vi "Modify Channel Test.vi"() -> (0 "no err":errorcluster, 3 "mod success":bool)   [LabVIEW 2017, in "ExampleStateMachine tests.lvlib"]
uses:
  ExampleStateMachine tests.lvlib
  <vilib>/NI/Tag Bus Module Framework/channel/TBM channel.lvclass/TBM channel.ctl
  <vilib>/NI/Tag Bus Module Framework/channel/channel classification.ctl
  <vilib>/NI/Tag Bus/tag/tag descriptor.lvclass/tag descriptor.ctl
  <vilib>/NI/Tag Bus Module Framework/channel/Read channel classification.vi
  <vilib>/NI/Tag Bus Module Framework/channel/Write channel classification.vi
  <vilib>/NI/Tag Bus Module Framework/channel/TBM channel.lvclass
  C:/Program Files (x86)/National Instruments/LabVIEW 2017/vi.lib/NI/Tag Bus/tag/tag descriptor.lvclass
  module/configuration/ExampleStateMachine configuration.lvclass
  <vilib>/NI/Tag Bus/tag/tag descriptor.lvclass
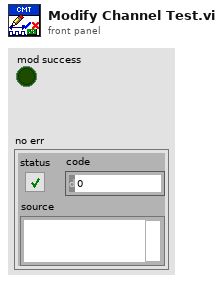
[diagram p1: front panel]
types:
  T1 = cluster{"channel":refnum<class "TBM channel.lvclass">}[]
  T2 = typedef "TBM channel.lvclass/channel classification.ctl" = enum16{"input data", "output data", "processing parameter", "processing result"}
  T3 = cluster{"channel":refnum<class "TBM channel.lvclass">}
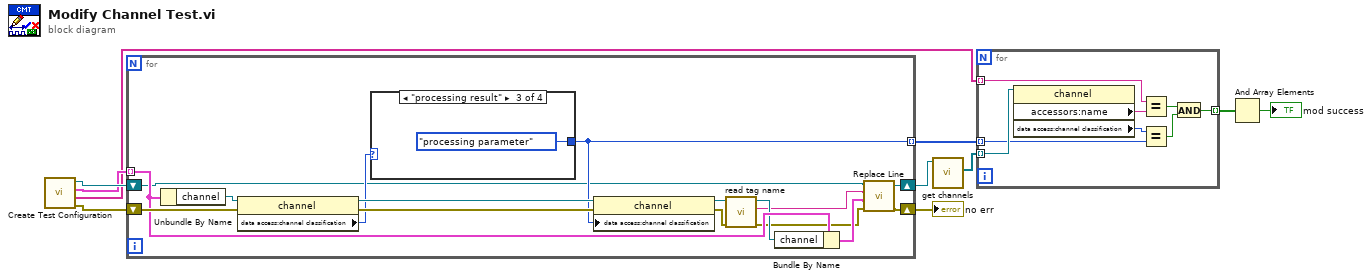
[diagram p0: block diagram]
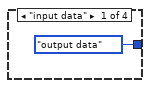
[diagram p2: hidden frame]
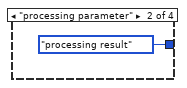
[diagram p3: hidden frame]
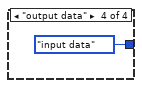
[diagram p4: hidden frame]
diagram:
  n1 = call "Create Test Configuration.vi"() -> ("error out"=w1:errorcluster, "Names"=w2:string[], "Line Array"=w3:T1, "Module"=w4:refnum<class "ExampleStateMachine configuration.lvclass">)  [unwired: 6 in, 2 out]
  n2 = for {
    shift-right: [w17] -> w10
    shift-left: w4 -> [w16]
    shift-right: [w13] -> w9
    shift-left: w1 -> [w26]
    tunnel: w3 -> [w20] mode=indexing
    tunnel: [w22] -> w5 mode=indexing
    n3 = Unbundle By Name(w20) -> ("channel"=w21:refnum<class "TBM channel.lvclass">)
    n4 = property class="channel"(reference=w21, error in=w26) -> (reference out=w24:refnum<class "TBM channel.lvclass">, error out=w25:errorcluster, "data access:channel classification"=w23:T2)
    n5 = case shown="\"processing result\"" w23 {
      tunnel: [channel_classification."output data" ("channel classification") channel_classification."processing result" ("channel classification") channel_classification."processing parameter" ("channel classification") channel_classification."input data" ("channel classification")] -> w22
      frame "input data" {
      }
      frame "processing parameter" {
      }
      frame "processing result" {
      }
      frame "output data" {
      }
    }
    n6 = property class="channel"(reference=w24, error in=w25, "data access:channel classification"=w22) -> (reference out=w19:refnum<class "TBM channel.lvclass">, error out=w11:errorcluster)
    n7 = call <vilib>:"read tag name.vi"("error in"=w11, "system tag in"=w19) -> ("error out"=w12:errorcluster, "name"=w15:string, "system tag out"=w18:refnum<class "TBM channel.lvclass">)  [unwired: 7 in]
    n8 = Bundle By Name(cluster=w20, "channel"=w18) -> (w14:T3)
    n9 = call-dynamic "Replace Line.vi"("error in (no error)"=w12, "New Line"=w14, "Line Name"=w15, "ExampleStateMachine configuration in"=w16) -> ("error out"=w13:errorcluster, "ExampleStateMachine configuration out"=w17:refnum<class "ExampleStateMachine configuration.lvclass">)  [unwired: 6 in]
  }
  "no err" <- w9
  n10 = call-dynamic "get channels.vi"("fixed channel configuration in"=w10) -> ("channels"=w8:refnum<class "TBM channel.lvclass">[])  [unwired: 9 in, 1 out]
  n11 = for {
    tunnel: w8 -> [w37] mode=indexing
    tunnel: [w36] -> w7 mode=indexing
    tunnel: w5 -> [w35] mode=indexing
    tunnel: w2 -> [w32] mode=indexing
    n12 = property class="channel"(reference=w37) -> ("accessors:name"=w33:string, "data access:channel classification"=w34:T2)  [unwired: 1 in, 2 out]
    n13 = Equal?(x=w32, y=w33) -> (x = y?=w31:bool)
    n14 = Equal?(x=w34, y=w35) -> (x = y?=w38:bool)
    n15 = And(x=w31, y=w38) -> (x .and. y?=w36:bool)
  }
  n16 = And Array Elements(Boolean array=w7) -> (logical AND=→"mod success":bool)
